vi "bmd101Parser_v0.vi"() -> ()   [LabVIEW 2016]
doc: "This example performs writes and reads on a serial port, as directed by the user. You can press the Write and Read buttons, and change the Read Count, while the example is running.\n\nThe parameters set for the serial port must match the parameters of the connected instrument or device. In this example, the Read Count parameter specifies the number of bytes that the serial port reads. If there were more bytes at the port than the specified number, those bytes would not be read. If there were less bytes at the port than the specified number, you would receive a timeout error.\n\nThis example expands upon the flow control options for XON and XOFF, allowing the user to choose those control characters. Also, the user can enable or disable a termination character. Some devices require a termination character in order to identify the end of command strings. Some devices send a termination character to signify the end of data to be read. This example shows how you can end the Read operation once a termination character is detected in the buffer and/or append a termination character at the end of the Write data."
uses:
  C:/Program Files/National Instruments/LabVIEW 2016/examples/Instrument IO/Serial/support/Serial - Settings.ctl
  <vilib>/Instr/_visa.llb/VISA Configure Serial Port (Instr).vi
panel:
  out "element":string
  out "packet conditions match?":bool
  out "packet=8byte?":bool
  out "Waveform Chart":i16[](graph)
  out "return count":u32
  out "Response":string
  in  "Read Count":u32=800
  in  "Read":bool=TRUE
  in  "Stop":bool
  in  "Serial Settings":T1={"baud rate"=57600, "data bits"=8, "parity"=enum."None", "stop bits"=10, "flow control"=0} {"flow control" items=["None"=0, "XON/XOFF"=1, "RTS/CTS"=2, "DTR/DSR"=4]; "stop bits" items=["1.0"=10, "1.5"=15, "2.0"=20]; "data bits" min=5 max=8 step=1; "baud rate" items=["75"=75, "110"=110, "134"=134, "150"=150, "300"=300, "600"=600, "1200"=1200, "1800"=1800, "2400"=2400, "4800"=4800, "7200"=7200, "9600"=9600, "14400"=14400, "19200"=19200, "28800"=28800, "38400"=38400, "56000"=56000, "57600"=57600, "115200"=115200, "128000"=128000, "230400"=230400]}
  in  "VISA resource name":refnum<visa-resource-name>="bmd101"
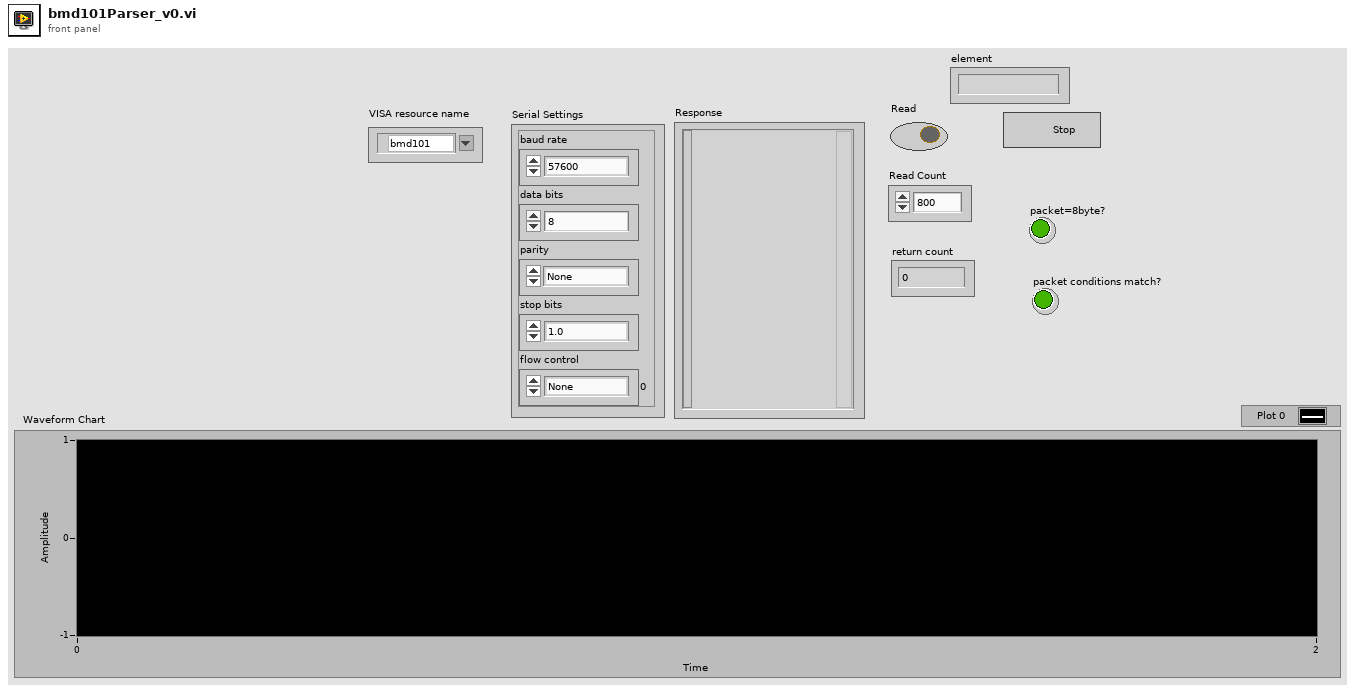
[diagram p1: front panel]
types:
  T1 = typedef "Serial - Settings.ctl" = cluster{"baud rate":u32, "data bits":u16, "parity":enum16{"None", "Odd", "Even", "Mark", "Space"}, "stop bits":u16, "flow control":u16}
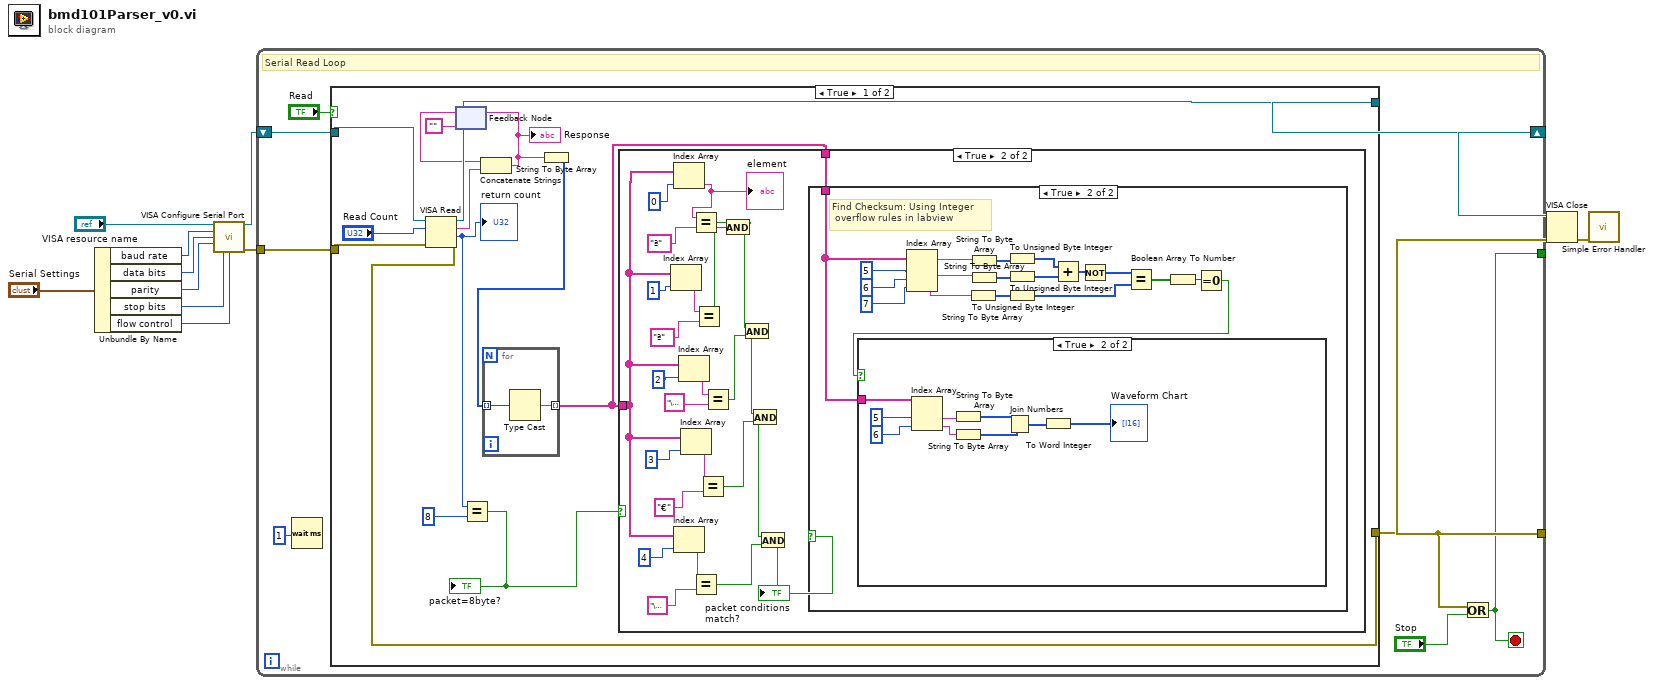
[diagram p0: block diagram]
diagram:
  n1 = Unbundle By Name("Serial Settings") -> ("baud rate"=w11:u32, "data bits"=w10:u16, "parity"=w9:enum16{"None", "Odd", "Even", "Mark", "Space"}, "stop bits"=w8:u16, "flow control"=w7:u16)
  n2 = call-poly "VISA Configure Serial Port"("VISA resource name"="VISA resource name", "baud rate (9600)"=w11, "data bits (8)"=w10, "parity (0:none)"=w9, "stop bits (10: 1 bit)"=w8, "flow control (0:none)"=w7) -> ("VISA resource name out"=w3:refnum<visa-resource-name>, "error out"=w2:errorcluster)  [unwired: 4 in, 4 out]
  n3 = while {
    shift-right: [w20] -> w4
    shift-left: w3 -> [w15]
    tunnel: w2 -> [w14]
    tunnel: [w17] -> w5
    tunnel: [w13] -> _
    stop <- w13 stop-if-true
    # "Serial Read Loop"
    n4 = Wait (ms)(milliseconds to wait=u32 1) -> ()  [unwired: 1 out]
    n5 = case shown="True" "Read" {
      tunnel: [w32 w91] -> w20
      tunnel: w15 -> [w34 w91]
      tunnel: [w30 w90] -> w17
      tunnel: w14 -> [w33 w90]
      frame True {
        n6 = VISA Read(VISA resource name=w34, byte count="Read Count", error in (no error)=w33) -> (VISA resource name out=w32:refnum<visa-resource-name>, read buffer=w29:string, return count=w24:u32, error out=w30:errorcluster)
        "return count" <- w24
        n7 = feedback #1("") -> (w28:string)
        n8 = Equal?(x=w24, y=8) -> (x = y?=w22:bool)
        "packet=8byte?" <- w22
        n9 = Concatenate Strings(w28, w29) -> (w25:string)
        "Response" <- w25
        n10 = feedback-in #1(w25) -> ()
        n11 = String To Byte Array(string=w25) -> (unsigned byte array=w26:u8[])
        n12 = for {
          tunnel: w26 -> [w89] mode=indexing
          tunnel: [w88] -> w21 mode=indexing
          n13 = Type Cast(x=w89) -> (*(type *) &x=w88:string)  [unwired: 1 in]
        }
        n14 = case shown="True" w22 {
          tunnel: w21 -> [_ w45]
          tunnel: w21 -> [_ w35]
          frame False {
          }
          frame True {
            n15 = Index Array(array=w45, index=1) -> (element=w55:string)
            n16 = Index Array(array=w45, index=0) -> (element=w59:string)
            "element" <- w59
            n17 = Index Array(array=w45, index=4) -> (element=w46:string)
            n18 = Index Array(array=w45, index=2) -> (element=w52:string)
            n19 = Index Array(array=w45, index=3) -> (element=w49:string)
            n20 = Equal?(x=w59, y="ª") -> (x = y?=w44:bool)
            n21 = Equal?(x=w46, y="\u0002") -> (x = y?=w37:bool)
            n22 = Equal?(x=w55, y="ª") -> (x = y?=w43:bool)
            n23 = Equal?(x=w49, y="€") -> (x = y?=w39:bool)
            n24 = Equal?(x=w52, y="\u0004") -> (x = y?=w41:bool)
            n25 = And(x=w44, y=w43) -> (x .and. y?=w42:bool)
            n26 = And(x=w42, y=w41) -> (x .and. y?=w40:bool)
            n27 = And(x=w40, y=w39) -> (x .and. y?=w38:bool)
            n28 = And(x=w38, y=w37) -> (x .and. y?=w36:bool)
            "packet conditions match?" <- w36
            n29 = case shown="True" w36 {
              tunnel: w35 -> [_ w61]
              frame False {
              }
              frame True {
                # "Find Checksum: Using Integer\n overflow rules in labview"
                n30 = Index Array(array=w61, index #1=5, index #2=6, index #3=7) -> (element #1=w76:string, element #2=w75:string, element #3=w68:string)
                n31 = String To Byte Array(string=w68) -> (unsigned byte array=w67:u8[])
                n32 = String To Byte Array(string=w76) -> (unsigned byte array=w73:u8[])
                n33 = String To Byte Array(string=w75) -> (unsigned byte array=w72:u8[])
                n34 = To Unsigned Byte Integer(number=w73) -> (unsigned 8bit integer=w71:u8[])
                n35 = To Unsigned Byte Integer(number=w72) -> (unsigned 8bit integer=w70:u8[])
                n36 = To Unsigned Byte Integer(number=w67) -> (unsigned 8bit integer=w65:u8[])
                n37 = Add(x=w71, y=w70) -> (x+y=w69:u8[])
                n38 = Not(x=w69) -> (.not. x?=w66:u8[])
                n39 = Equal?(x=w66, y=w65) -> (x = y?=w64:bool[])
                n40 = Boolean Array To Number(Boolean array=w64) -> (number=w63:u32)
                n41 = Equal To 0?(x=w63) -> (x = 0?=w62:bool)
                n42 = case shown="True" w62 {
                  tunnel: w61 -> [_ w87]
                  frame False {
                  }
                  frame True {
                    n43 = Index Array(array=w87, index #1=5, index #2=6) -> (element #1=w84:string, element #2=w83:string)
                    n44 = String To Byte Array(string=w84) -> (unsigned byte array=w82:u8[])
                    n45 = String To Byte Array(string=w83) -> (unsigned byte array=w81:u8[])
                    n46 = Join Numbers(hi=w82, lo=w81) -> ((hi.lo)=w80:u16[])
                    n47 = To Word Integer(number=w80) -> (16bit integer=→"Waveform Chart":i16[])
                  }
                }
              }
            }
          }
        }
      }
      frame False {
      }
    }
    n48 = Or(x=w17, y="Stop") -> (x .or. y?=w13:bool)
  }
  n49 = VISA Close(VISA resource name=w4, error in (no error)=w5) -> (error out=w1:errorcluster)
  n50 = call <vilib>:"Simple Error Handler.vi"("error in (no error)"=w1) -> ()  [unwired: 1 in, 8 out]
